vi "3-7.vi"   [LabVIEW 2022 SP3]
uses:
  <vilib>/Utility/file.llb/Write Delimited Spreadsheet (DBL).vi
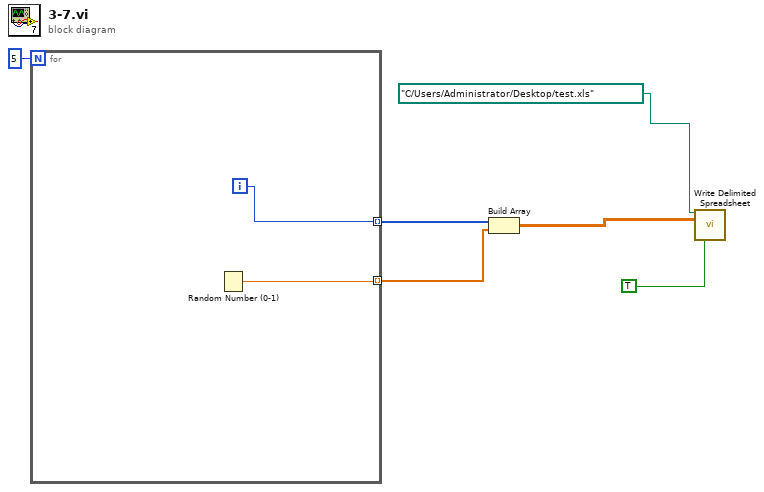
[diagram p0: block diagram]
diagram:
  n1 = for {
    N: 5 -> [_]
    tunnel: [w8] -> w5 mode=indexing
    tunnel: [w7] -> w4 mode=indexing
    i -> [w8]
    n2 = Random Number (0-1)() -> (number: 0 to 1=w7:dbl)
  }
  n3 = Build Array(w5, w4) -> (w3:dbl[][])
  n4 = call-poly <vilib>:"Write Delimited Spreadsheet.vi"("file path (dialog if empty)"=path "C:/Users/Administrator/Desktop/test.xls", "2D data"=w3, "transpose? (no:F)"=TRUE) -> ()  [unwired: 11 in, 2 out]
